vi "Pareto PDF.vi"(9 "c":dbl=3.0, 10 "a":dbl=1.0, 11 "x":dbl=2.0) -> (0 "error":i32, 3 "pdf(x)":dbl=0.1875)   [LabVIEW 2014, in "NI_Gmath.lvlib"]
doc: "Computes the continuous probability density function (PDF) of various distributions. You must manually select the polymorphic instance to use."
uses:
  NI_Gmath.lvlib
  st_error_code.ctl
panel:
  # "Pareto PDF"
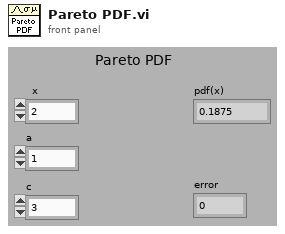
[diagram p1: front panel]
types:
  T1 = typedef "NI_Gmath.lvlib/st_error_code.ctl" = i32
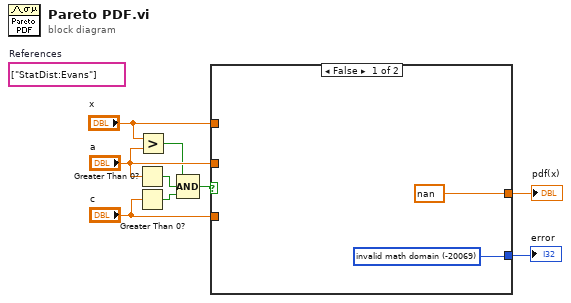
[diagram p0: block diagram]
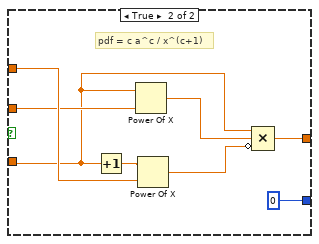
[diagram p2: hidden frame]
diagram:
  (unwired) string[] ["StatDist:Evans"]  # References
  n1 = Greater Than 0?(x="a") -> (x > 0?=w3:bool)
  n2 = Greater Than 0?(x="c") -> (x > 0?=w2:bool)
  n3 = Greater?(x="x", y="a") -> (0:w4:bool)
  n4 = Compound Arithmetic op=AND(w4, w3, w2) -> (w1:bool)
  n5 = case shown="False" w1 {
    tunnel: "c" -> [_ w14]
    tunnel: [w10 0 ("invalid math domain")] -> w9
    tunnel: [nan w18] -> w8
    tunnel: "x" -> [_ w17]
    tunnel: "a" -> [_ w15]
    frame False {
      w10 = T1 -20069 items=["invalid math domain"=-20069, "Fourier interpolation size m >= n"=-20070, "empty array"=-20003] ("stat interp error code")
    }
    frame True {
      # "pdf = c a^c / x^(c+1)"
      n6 = Increment(x=w14) -> (x+1=w16:dbl)
      n7 = Power Of X(1:w15, 2:w14) -> (0:w13:dbl)
      n8 = Power Of X(1:w17, 2:w16) -> (0:w12:dbl)
      n9 = Compound Arithmetic op=MULTIPLY(w14, w13, invert w12) -> (w18:dbl)
    }
  }
  "pdf(x)" <- w8
  "error" <- w9
